vi "Unmap Memory.vi"(8 "error in (no error)":errorcluster, 11 "Shared Memory in":refnum<class "Shared Memory.lvclass">) -> (0 "error out":errorcluster, 3 "Shared Memory out":refnum<class "Shared Memory.lvclass">)   [LabVIEW 2016, in "Linux RT IPC.Shared Memory.lvlib" / "Shared Memory.lvclass"]
doc: "This VI calls the munmap() function which unmaps the shared memory resource from the calling processes memory space."
uses:
  Shared Memory.lvclass
  Shared Memory.lvclass/Shared Memory.ctl
  C/SubVIs/error handler.vi
  <vilib>/NI/NI Linux RT Errno/VIs/Public/Get Errno Value for Calling Thread.vi
  C/Linux RT IPC.C.lvlib
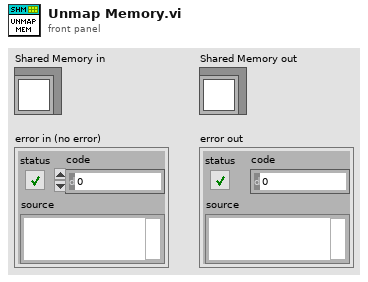
[diagram p1: front panel]
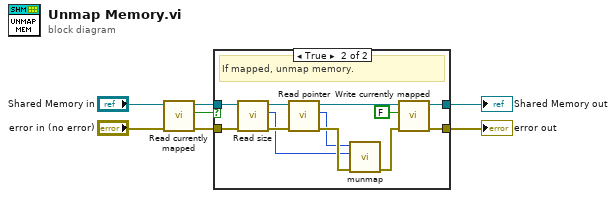
[diagram p0: block diagram]
diagram:
  n1 = call "Read currently mapped.vi"("error in (no error)"="error in (no error)", "Shared Memory in"="Shared Memory in") -> ("error out"=w4:errorcluster, "currently mapped"=w5:bool, "Shared Memory out"=w3:refnum<class "Shared Memory.lvclass">)  [unwired: 7 in]
  n2 = case shown="True" w5 {
    tunnel: [w8 w12] -> w6
    tunnel: w3 -> [w8 w19]
    tunnel: w4 -> [w9 w18]
    tunnel: [w9 w13] -> w7
    frame False {
      # "Not mapped. Do nothing."
    }
    frame True {
      # "If mapped, unmap memory."
      n3 = call "Read size.vi"("error in (no error)"=w18, "Shared Memory in"=w19) -> ("error out"=w17:errorcluster, "size (bytes)"=w15:u64, "Shared Memory out"=w16:refnum<class "Shared Memory.lvclass">)  [unwired: 7 in]
      n4 = call "Read pointer.vi"("error in (no error)"=w17, "Shared Memory in"=w16) -> ("error out"=w21:errorcluster, "pointer"=w20:u64, "Shared Memory out"=w14:refnum<class "Shared Memory.lvclass">)  [unwired: 7 in]
      n5 = call "munmap.vi"("error in (no error)"=w21, "size (bytes)"=w15, "pointer"=w20) -> ("error out"=w10:errorcluster)  [unwired: 8 in]
      n6 = call "Write currently mapped.vi"("error in (no error)"=w10, "currently mapped"=FALSE, "Shared Memory in"=w14) -> ("error out"=w13:errorcluster, "Shared Memory out"=w12:refnum<class "Shared Memory.lvclass">)  [unwired: 7 in]
    }
  }
  "error out" <- w7
  "Shared Memory out" <- w6
